vi "Initialize.vi"(8 "error in (no error)":errorcluster, 10 "Reply to":refnum<class "Result Reply Msg.lvclass">, 11 "Measure Controller in":refnum<class "Measure Controller.lvclass">) -> (0 "error out":errorcluster, 3 "Measure Controller out":refnum<class "Measure Controller.lvclass">)   [LabVIEW 2015, in "Measure Controller.lvclass"]
uses:
  Measure Controller.lvclass
  Measure Object Messages/Result Reply Msg/Result Reply Msg.lvclass
  Measure Controller Messages/Init Response Msg/Init Response Msg.lvclass
  Results/Acquired Result/Acquired Result.lvclass
  Measure Object Messages/Initialize Msg/Initialize Msg.lvclass/Initialize Msg.ctl
  <vilib>/ActorFramework/Message Enqueuer/Message Enqueuer.lvclass/Message Enqueuer.ctl
  Measure Controller.lvclass/Measure Controller.ctl
  <vilib>/ActorFramework/Message Enqueuer/Enqueue.vi
  <vilib>/ActorFramework/Message Priority Queue/Priority Enqueue.vi
  Measure Object Messages/Initialize Msg/Initialize Msg.lvclass
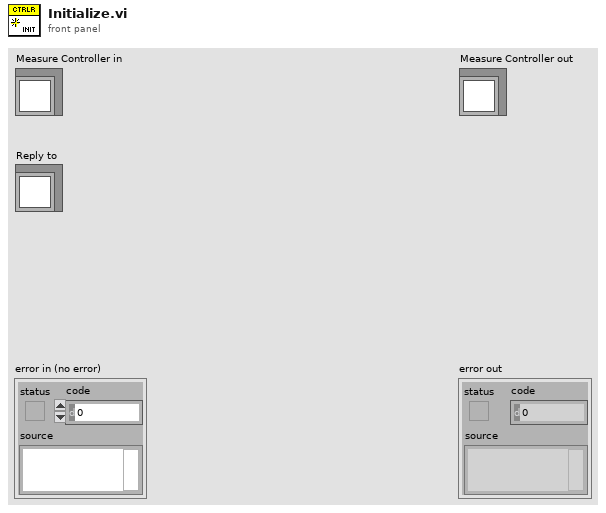
[diagram p1: front panel]
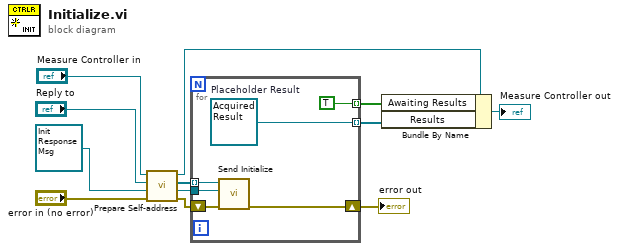
[diagram p0: block diagram]
diagram:
  n1 = call-dynamic "Prepare Self-address.vi"("error in (no error)"="error in (no error)", "Reply to me"=refnum<class "Init Response Msg.lvclass"> refnum ("Init Response Msg.lvclass"), "Reply to"="Reply to", "Measure Controller in"="Measure Controller in") -> ("error out"=w4:errorcluster, "Reply to me"=w7:refnum<class "Result Reply Msg.lvclass">, "Active measurements enqueuers"=w6:refnum<class "Message Enqueuer.lvclass">[], "Measure Controller out"=w2:refnum<class "Measure Controller.lvclass">)  [unwired: 4 in]
  n2 = for {
    tunnel: w6 -> [w14] mode=indexing
    shift-right: [w18] -> w9
    shift-left: w4 -> [w13]
    tunnel: [TRUE] -> w12 mode=indexing
    tunnel: [w16] -> w11 mode=indexing
    tunnel: w7 -> [w15]
    w16 = refnum<class "Acquired Result.lvclass"> refnum  # Placeholder Result
    n3 = call "Send Initialize.vi"("error in (no error)"=w13, "Reply to"=w15, "Message Enqueuer"=w14) -> ("error out"=w18:errorcluster)  [unwired: 7 in, 1 out]
  }
  "error out" <- w9
  n4 = Bundle By Name(cluster=w2, "Awaiting Results"=w12, "Results"=w11) -> (→"Measure Controller out":refnum<class "Measure Controller.lvclass">)
